vi "publish_C1_ACS_status.vi"() -> ()   [LabVIEW 2018]
uses:
  RxTx/CCS_RxTx.lvclass
  <vilib>/addons/zeromq/socket_type.ctl
  <vilib>/addons/zeromq/zmq_socket.lvclass
  <vilib>/addons/zeromq/zmq_context.lvclass
  <vilib>/addons/zeromq/zeromq.lvlib
panel:
  in  "Stop Button":bool
  out "error out":errorcluster
  out "error out 3":errorcluster
  in  "RxTx.lvclass 2":refnum<class "CCS_RxTx.lvclass">
  # "Channel 1 - ZEROMQ Communication"
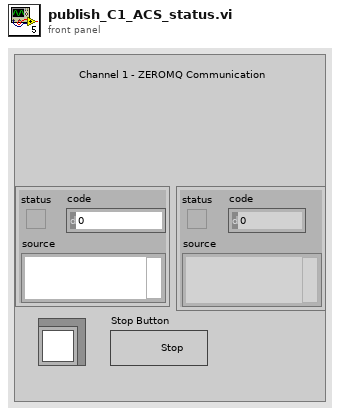
[diagram p1: front panel]
types:
  T1 = typedef "zeromq.lvlib/socket_type.ctl" = enum8{"ZMQ_PAIR", "ZMQ_PUB", "ZMQ_SUB", "ZMQ_REQ", "ZMQ_REP", "ZMQ_DEALER", "ZMQ_ROUTER", "ZMQ_PULL", "ZMQ_PUSH", "ZMQ_XPUB", "ZMQ_XSUB", "ZMQ_STREAM", "ZMQ_SERVER", "ZMQ_CLIENT", "ZMQ_RADIO", "ZMQ_DISH", "ZMQ_GATHER", "ZMQ_SCATTER", "ZMQ_DGRAM"}
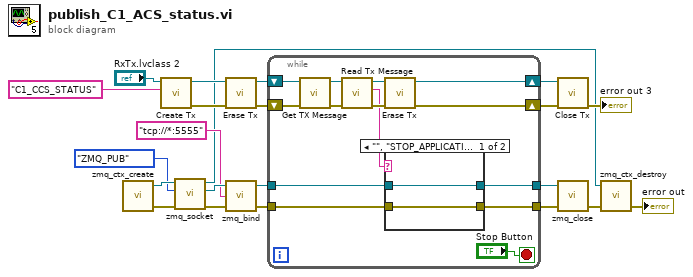
[diagram p0: block diagram]
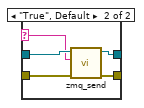
[diagram p2: hidden frame]
diagram:
  n1 = call <vilib>:"zmq_ctx_create.vi"() -> ("error out"=w11:errorcluster, "context out"=w14:refnum<class "zmq_context.lvclass">)  [unwired: 4 in]
  n2 = call "Create Tx.vi"("Writer Name"="C1_CCS_STATUS" ("string"), "RxTx in"="RxTx.lvclass 2") -> ("error out"=w18:errorcluster, "RxTx out"=w19:refnum<class "CCS_RxTx.lvclass">)  [unwired: 8 in]
  n3 = call <vilib>:"zmq_socket.vi"("error in"=w11, "socket type"=socket_type."ZMQ_PUB", "context in"=w14) -> ("error out"=w13:errorcluster, "socket out"=w12:refnum<class "zmq_socket.lvclass">, "context out"=w5:refnum<class "zmq_context.lvclass">)  [unwired: 2 in]
  n4 = call "Erase Tx.vi"("error in (no error)"=w18, "RxTx in"=w19) -> ("error out"=w15:errorcluster, "RxTx out"=w17:refnum<class "CCS_RxTx.lvclass">)  [unwired: 8 in]
  n5 = call <vilib>:"zmq_bind.vi"("error in"=w13, "endpoint"="tcp://*:5555", "socket in"=w12) -> ("error out"=w6:errorcluster, "socket out"=w7:refnum<class "zmq_socket.lvclass">)  [unwired: 1 in]
  n6 = while {
    shift-right: [w36] -> w22
    shift-left: w17 -> [w31]
    shift-right: [w29] -> w16
    shift-left: w15 -> [w30]
    tunnel: w7 -> [w28]
    tunnel: w6 -> [w27]
    tunnel: [w26] -> w4
    tunnel: [w25] -> w3
    stop <- "Stop Button" stop-if-true
    n7 = call "Get TX Message.vi"("error in (no error)"=w30, "RxTx in"=w31) -> ("error out"=w35:errorcluster, "RxTx out"=w32:refnum<class "CCS_RxTx.lvclass">)  [unwired: 8 in]
    n8 = call "Read Tx Message.vi"("error in (no error)"=w35, "RxTx in"=w32) -> ("error out"=w33:errorcluster, "Tx Message"=w24:string, "RxTx out"=w34:refnum<class "CCS_RxTx.lvclass">)  [unwired: 7 in]
    n9 = call "Erase Tx.vi"("error in (no error)"=w33, "RxTx in"=w34) -> ("error out"=w29:errorcluster, "RxTx out"=w36:refnum<class "CCS_RxTx.lvclass">)  [unwired: 8 in]
    n10 = case shown="\"\", \"STOP_APPLICATION\"" w24 {
      selector: w24 -> [_ w39]
      tunnel: w28 -> [w38 w43]
      tunnel: w27 -> [w37 w42]
      tunnel: [w38 w41] -> w26
      tunnel: [w37 w40] -> w25
      frame "", "STOP_APPLICATION" {
      }
      frame "True", Default {
        n11 = call <vilib>:"zmq_send.vi"("error in"=w42, "data"=w39, "socket in"=w43) -> ("error out"=w40:errorcluster, "socket out"=w41:refnum<class "zmq_socket.lvclass">)  [unwired: 4 in]
      }
    }
  }
  n12 = call "Close Tx.vi"("error in (no error)"=w16, "RxTx in"=w22) -> ("error out"=→"error out 3":errorcluster)  [unwired: 8 in, 1 out]
  n13 = call <vilib>:"zmq_close.vi"("error in"=w3, "socket"=w4) -> ("error out"=w8:errorcluster)  [unwired: 3 in]
  n14 = call <vilib>:"zmq_ctx_destroy.vi"("error in"=w8, "context in"=w5) -> ("error out"=→"error out":errorcluster)  [unwired: 3 in]
